vi "Auto Set Camera Settings.vi"(11 "Run?":bool) -> (3 "Done":bool)   [LabVIEW 2013]
uses:
  <vilib>/Rock Robotics/WPI/Camera/WPI_CameraWhite Balance Values.ctl
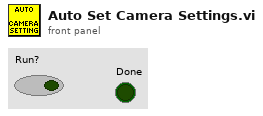
[diagram p1: front panel]
types:
  T1 = typedef "WPI_CameraWhite Balance Values.ctl" = enum16{"Auto", "Fixed indoor", "Fixed outdoor 1", "Fixed outdoor 2", "Fixed fluorescent 1", "Fixed fluorescent 2", "Hold current"}
  T2 = typedef "WPI_CameraDevRef.ctl" = cluster{"Camera Address":string, "CameraStatus":errorcluster, "Acquire Image Notifier":refnum<notifier>}
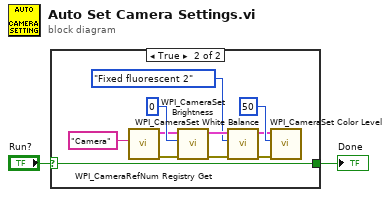
[diagram p0: block diagram]
diagram:
  n1 = case shown="True" "Run?" {
    selector: "Run?" -> [w3 w7]
    tunnel: [w3 w7] -> w1
    frame False {
    }
    frame True {
      n2 = call <vilib>:"WPI_CameraRefNum Registry Get.vi"("refnum name"="Camera") -> ("error out"=w5:errorcluster, "CameraDevRef"=w6:T2)  [unwired: 9 in]
      n3 = call <vilib>:"WPI_CameraSet Brightness.vi"("error in (no error)"=w5, "Brightness"=0, "CameraDevRef"=w6) -> ("error out"=w11:errorcluster, "CameraDevRef Out"=w14:T2)  [unwired: 7 in]
      n4 = call <vilib>:"WPI_CameraSet White Balance.vi"("error in (no error)"=w11, "White Balance"=WPI_CameraWhite_Balance_Values."Fixed fluorescent 2", "CameraDevRef"=w14) -> ("error out"=w10:errorcluster, "CameraDevRef Out"=w8:T2)  [unwired: 7 in]
      n5 = call <vilib>:"WPI_CameraSet Color Level.vi"("error in (no error)"=w10, "Color Level"=50, "CameraDevRef"=w8) -> ()  [unwired: 7 in, 2 out]
    }
  }
  "Done" <- w1
